vi "_FPGA_U32equal2.vi"(10 "Numeric":u32) -> (2 "==2?":bool)   [LabVIEW 2018]
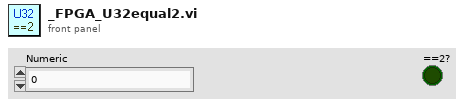
[diagram p1: front panel]
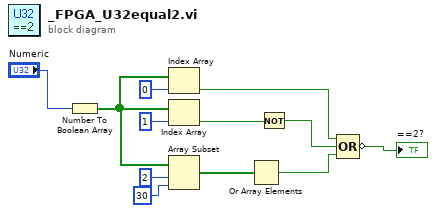
[diagram p0: block diagram]
diagram:
  n1 = Number To Boolean Array(number="Numeric") -> (Boolean array=w3:bool[])
  n2 = Index Array(array=w3, index=0) -> (element=w1:bool)
  n3 = Index Array(array=w3, index=1) -> (element=w8:bool)
  n4 = Array Subset(array=w3, index=2, length=30) -> (w7:bool[])
  n5 = Or Array Elements(Boolean array=w7) -> (logical OR=w5:bool)
  n6 = Not(x=w8) -> (.not. x?=w6:bool)
  n7 = Compound Arithmetic op=OR(w1, w6, w5) -> (invert →"==2?":bool)
